vi "Extract spectrum.vi"(2 "Spectrum ref":refnum<vi>, 3 "Bins Cluster":cluster{"Max":dbl, "Min":dbl, "# bins":i32}, 4 "Spectrum Data":T3, 5 "Integral Spectrum":dbl[][](array[numeric]), 6 "Peak Vs Integral":bool, 7 "File Vs Discr.":bool) -> (0 "Nb of Counts":T2, 1 "Spectrum Histogram":T1(graph))   [LabVIEW 2019]
uses:
  ESA_Data_Analysis_Global_VIs.vi
  <vilib>/Analysis/NI_AALPro.lvlib
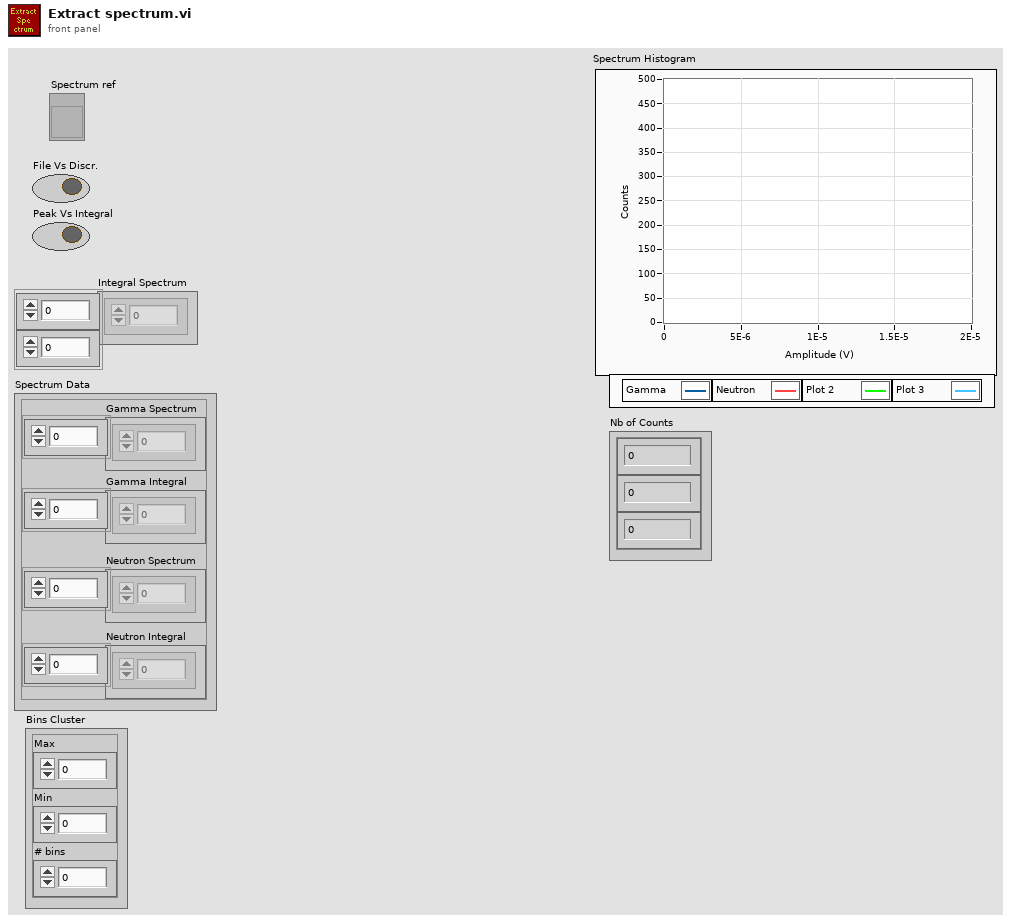
[diagram p1: front panel]
types:
  T1 = cluster{"X Values":dbl[], "Histogram: h(x)":i32[]}[]
  T2 = cluster{"Numeric Control":i32, "Numeric Control":i32, "Numeric Control":i32}
  T3 = cluster{"Gamma Spectrum":dbl[], "Gamma Integral":dbl[], "Neutron Spectrum":dbl[], "Neutron Integral":dbl[]}
  T4 = cluster{"X Values":dbl[], "Histogram: h(x)":i32[]}
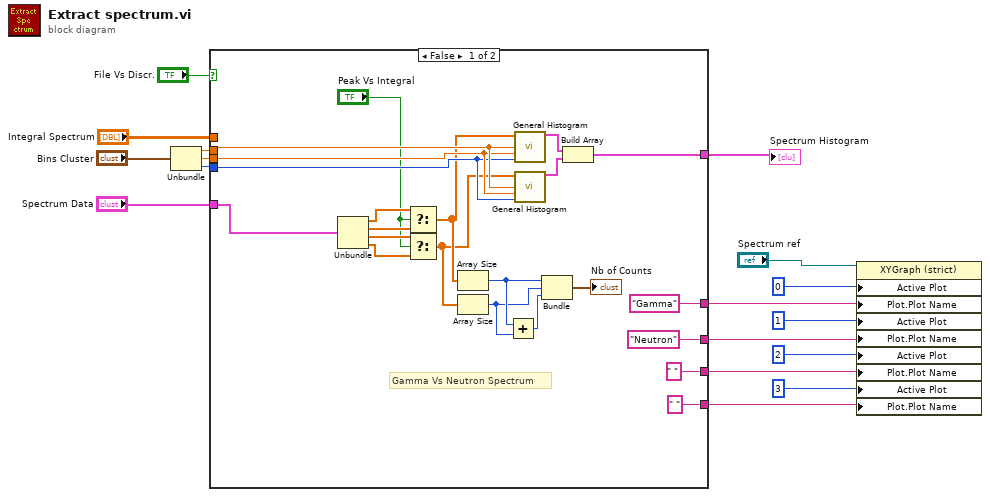
[diagram p0: block diagram]
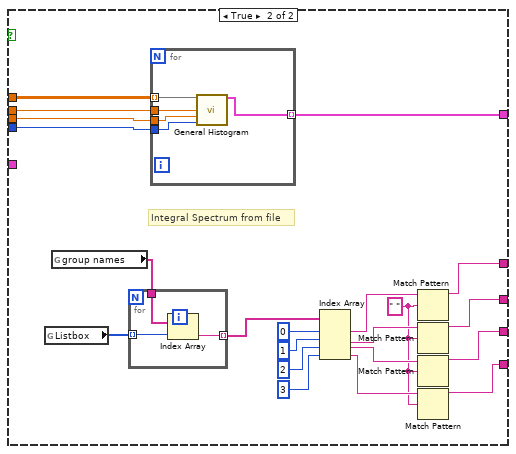
[diagram p2: hidden frame]
diagram:
  n1 = Unbundle("Bins Cluster") -> ("Max"=w13:dbl, "Min"=w12:dbl, "# bins"=w11:i32)
  n2 = case shown="False" "File Vs Discr." {
    tunnel: "Integral Spectrum" -> [_ w60]
    tunnel: w13 -> [w38 w59]
    tunnel: w12 -> [w37 w58]
    tunnel: w11 -> [w36 w57]
    tunnel: [w28 w56] -> w10
    tunnel: "Spectrum Data" -> [w39 _]
    tunnel: ["Gamma" ("Plot.Plot Name") w50] -> w8
    tunnel: ["Neutron" ("Plot.Plot Name") w45] -> w6
    tunnel: [" " ("Plot.Plot Name") w44] -> w2
    tunnel: [" " ("Plot.Plot Name") w43] -> w1
    frame False {
      # "Gamma Vs Neutron Spectrum"
      n3 = Unbundle(w39) -> ("Gamma Spectrum"=w33:dbl[], "Gamma Integral"=w32:dbl[], "Neutron Spectrum"=w31:dbl[], "Neutron Integral"=w30:dbl[])
      n4 = Select(t=w33, s="Peak Vs Integral", f=w32) -> (s? t:f=w27:dbl[])
      n5 = Select(t=w31, s="Peak Vs Integral", f=w30) -> (s? t:f=w26:dbl[])
      n6 = Array Size(array=w27) -> (size(s)=w25:i32)
      n7 = Array Size(array=w26) -> (size(s)=w24:i32)
      n8 = Add(x=w25, y=w24) -> (x+y=w23:i32)
      n9 = call <vilib>:"General Histogram.vi"("X"=w27, "max"=w38, "min"=w37, "# bins"=w36) -> ("Histogram Graph"=w34:T4)  [unwired: 7 in, 4 out]
      n10 = call <vilib>:"General Histogram.vi"("X"=w26, "max"=w38, "min"=w37, "# bins"=w36) -> ("Histogram Graph"=w35:T4)  [unwired: 7 in, 4 out]
      n11 = Bundle(w25, w24, w23) -> (→"Nb of Counts":cluster{i32, i32, i32})  [unwired: 1 in]
      n12 = Build Array(w34, w35) -> (w28:T1)
    }
    frame True {
      w46 = " " ("regular expression")
      # "Integral Spectrum from file"
      n13 = global read "ESA_Data_Analysis_Global_VIs.vi" "Listbox"() -> (w42:i32[])
      n14 = global read "ESA_Data_Analysis_Global_VIs.vi" "group names"() -> (w41:string[])
      n15 = for {
        tunnel: w42 -> [w62] mode=indexing
        tunnel: w41 -> [w63]
        tunnel: [w61] -> w40 mode=indexing
        n16 = Index Array(array=w63, index=w62) -> (element=w61:string)
      }
      n17 = for {
        tunnel: w60 -> [w68] mode=indexing
        tunnel: w59 -> [w67]
        tunnel: w58 -> [w66]
        tunnel: w57 -> [w65]
        tunnel: [w64] -> w56 mode=indexing
        n18 = call <vilib>:"General Histogram.vi"("X"=w68, "max"=w67, "min"=w66, "# bins"=w65) -> ("Histogram Graph"=w64:T4)  [unwired: 7 in, 4 out]
      }
      n19 = Index Array(array=w40, index #1=0 ("index"), index #2=1 ("index"), index #3=2 ("index"), index #4=3 ("index")) -> (element #1=w51:string, element #2=w49:string, element #3=w48:string, element #4=w47:string)
      n20 = Match Pattern(string=w51, regular expression=w46) -> (before substring=w50:string)  [unwired: 1 in, 3 out]
      n21 = Match Pattern(string=w49, regular expression=w46) -> (before substring=w45:string)  [unwired: 1 in, 3 out]
      n22 = Match Pattern(string=w48, regular expression=w46) -> (before substring=w44:string)  [unwired: 1 in, 3 out]
      n23 = Match Pattern(string=w47, regular expression=w46) -> (before substring=w43:string)  [unwired: 1 in, 3 out]
    }
  }
  "Spectrum Histogram" <- w10
  n24 = property class="XYGraph (strict)"(reference="Spectrum ref", "Active Plot"=u32 0, "Plot.Plot Name"=w8, "Active Plot"=u32 1, "Plot.Plot Name"=w6, "Active Plot"=u32 2, "Plot.Plot Name"=w2, "Active Plot"=u32 3, "Plot.Plot Name"=w1) -> ()  [unwired: 1 in, 2 out]
